vi "Read Data Model.vi"(8 "error in":errorcluster, 11 "Modbus slave in":refnum<class "Modbus Slave.lvclass">) -> (0 "error out":errorcluster, 2 "Device Data Model":refnum<class "Device Data Model.lvclass">, 3 "Modbus slave out":refnum<class "Modbus Slave.lvclass">)   [LabVIEW 2012, in "Modbus Slave.lvclass"]
doc: "This VI is an accessor for the <B>data model</B> stored in the Modbus master instance. This accessor can be used as a property node. This model defines how the slave stores data and reacts to functions and data sent by a Modbus master."
uses:
  Modbus Slave.lvclass
  Data Model/Device Data Model.lvclass
  Modbus Slave.lvclass/Modbus Slave.ctl
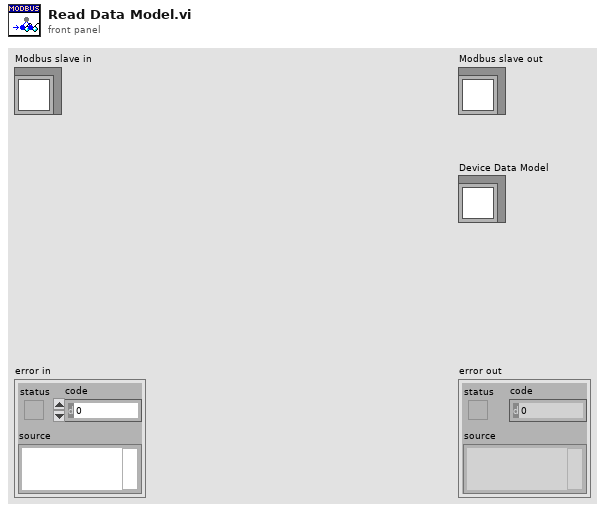
[diagram p1: front panel]
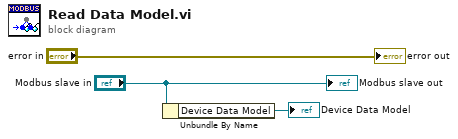
[diagram p0: block diagram]
diagram:
  n1 = Unbundle By Name("Modbus slave in") -> ("Device Data Model"=→"Device Data Model":refnum<class "Device Data Model.lvclass">)
  "error out" <- "error in"
  "Modbus slave out" <- "Modbus slave in"
